vi "Motor_FeedforwardVol.vi"(8 "error in (no error)":errorcluster, 10 "TensionRef":dbl[](array[numeric]), 11 "Motors_New in":refnum<class "MotorControl.lvclass">) -> (0 "error out":errorcluster, 2 "FeedForwardVol":dbl[](array[numeric]), 3 "Motors_New out":refnum<class "MotorControl.lvclass">)   [LabVIEW 2015, in "MotorControl.lvclass"]
uses:
  MotorControl.lvclass
  MotorControl.lvclass/MotorControl.ctl
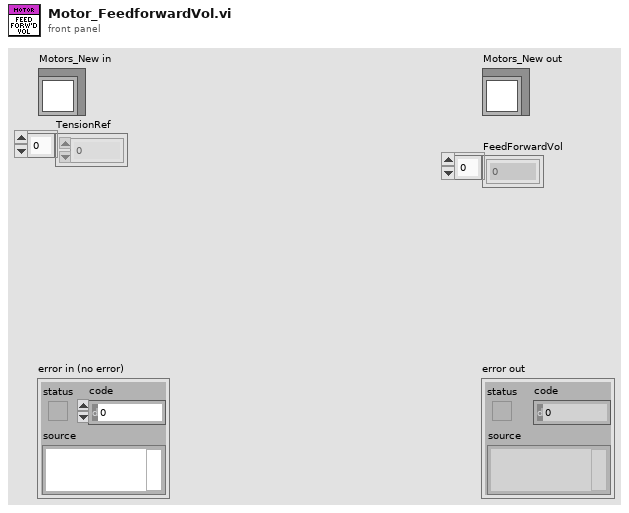
[diagram p1: front panel]
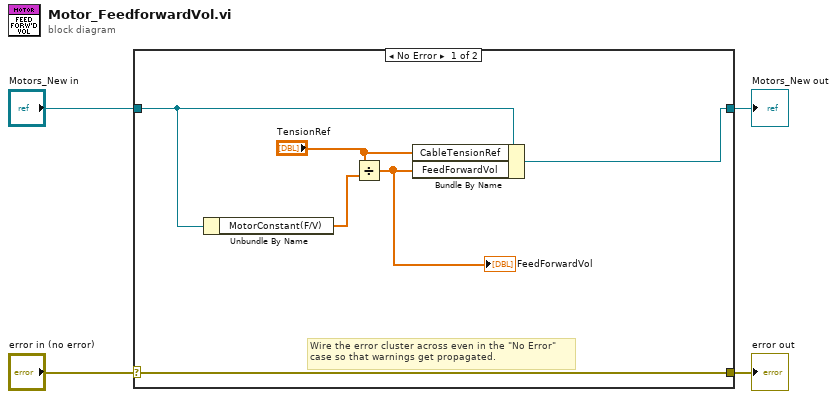
[diagram p0: block diagram]
diagram:
  n1 = case shown="No Error" "error in (no error)" {
    selector: "error in (no error)" -> [w10 w12]
    tunnel: [w10 w12] -> w3
    tunnel: [w6 w11] -> w1
    tunnel: "Motors_New in" -> [w7 w11]
    frame No Error {
      # "Wire the error cluster across even in the \"No Error\"\ncase so that warnings get propagated."
      n2 = Unbundle By Name(w7) -> ("MotorConstant(F/V)"=w9:dbl[])
      n3 = Divide(x="TensionRef", y=w9) -> (x/y=w8:dbl[])
      "FeedForwardVol" <- w8
      n4 = Bundle By Name(cluster=w7, "CableTensionRef"="TensionRef", "FeedForwardVol"=w8) -> (w6:refnum<class "MotorControl.lvclass">)
    }
    frame Error {
    }
  }
  "error out" <- w3
  "Motors_New out" <- w1
